vi "Nested Object Stopped.vi"(8 "error in (no error)":errorcluster, 10 "Name":string, 11 "Mag Lab Measure Base in":refnum<class "Mag Lab Measure Base.lvclass">) -> (0 "error out":errorcluster, 3 "Mag Lab Measure Base out":refnum<class "Mag Lab Measure Base.lvclass">)   [LabVIEW 2015, in "Mag Lab Measure Base.lvclass"]
uses:
  Mag Lab Measure Base.lvclass
  Mag Lab Measure Base.lvclass/Mag Lab Measure Base.ctl
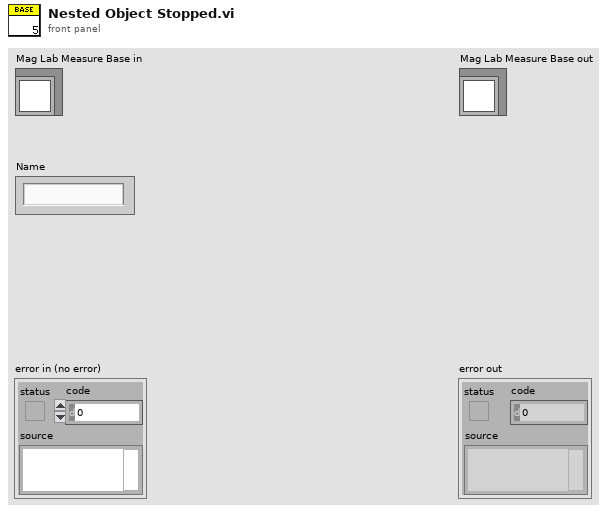
[diagram p1: front panel]
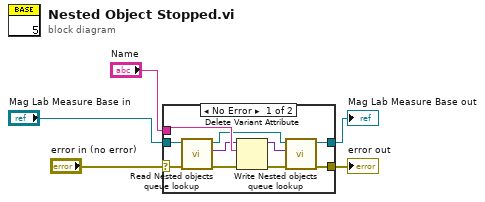
[diagram p0: block diagram]
diagram:
  n1 = case shown="No Error" "error in (no error)" {
    selector: "error in (no error)" -> [w13 w17]
    tunnel: [w7 w17] -> w4
    tunnel: [w9 w16] -> w2
    tunnel: "Mag Lab Measure Base in" -> [w15 w16]
    tunnel: "Name" -> [w14 _]
    frame No Error {
      n2 = call "Read Nested objects queue lookup.vi"("error in (no error)"=w13, "Mag Lab Measure Base in"=w15) -> ("error out"=w12:errorcluster, "Nested objects queue lookup"=w11:variant, "Mag Lab Measure Base out"=w10:refnum<class "Mag Lab Measure Base.lvclass">)  [unwired: 7 in]
      n3 = Delete Variant Attribute(4:w12, 6:w14, 7:w11) -> (0:w8:errorcluster, 3:w6:variant)  [unwired: 1 out]
      n4 = call "Write Nested objects queue lookup.vi"("error in (no error)"=w8, "Nested objects queue lookup"=w6, "Mag Lab Measure Base in"=w10) -> ("error out"=w7:errorcluster, "Mag Lab Measure Base out"=w9:refnum<class "Mag Lab Measure Base.lvclass">)  [unwired: 7 in]
    }
    frame Error {
    }
  }
  "error out" <- w4
  "Mag Lab Measure Base out" <- w2
